vi "Example Read File.vi"() -> ()   [LabVIEW 2013]
uses:
  C:/tf/play/labview/Tinkerforge.dll
  Tinkerforge.dll
panel:
  out "transferred (byte)":i32
  in  "local path":path=path "C:/foobar.txt"
  in  "remote path":string="/home/tf/foobar.txt"
  in  "uid":string="XXYYZZ"
  in  "port":i32=4223
  in  "host":string="localhost"
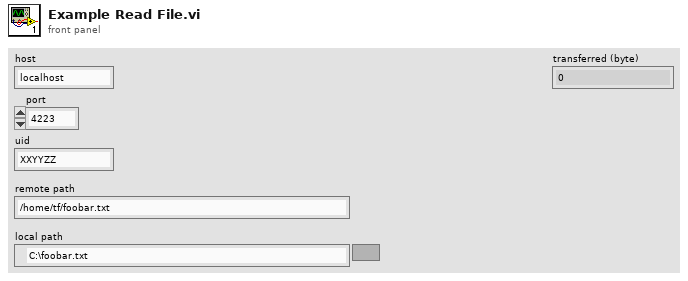
[diagram p1: front panel]
types:
  T1 = enum16{"open", "replace", "create", "open or create", "replace or create", "replace or create with confirmation"}
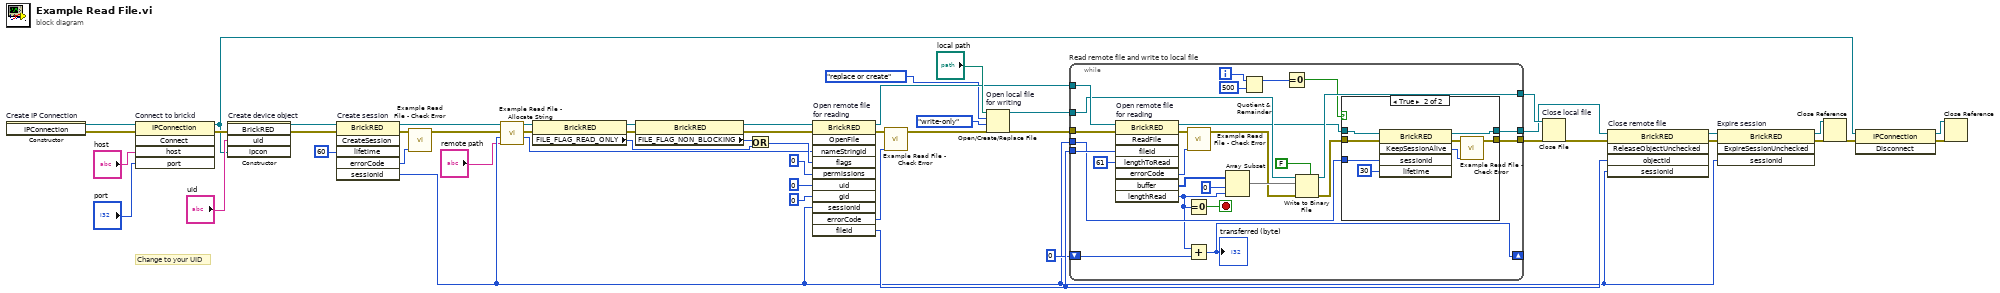
[diagram p0: block diagram]
diagram:
  # "Change to your UID"
  n1 = constructor on="Create IP Connection" class="IPConnection"() -> (reference out=w51:refnum<k24>, error out=w40:errorcluster)  [unwired: 3 in, 1 out]
  n2 = invoke on="Connect to brickd" class="IPConnection" method="Connect"(reference=w51, error in=w40, "host"="host", "port"="port") -> (reference out=w42:refnum<k24>, error out=w47:errorcluster)  [unwired: 1 in, 3 out]
  n3 = constructor on="Create device object" class="BrickRED"(error in=w47, "uid"="uid", "ipcon"=w42) -> (reference out=w45:refnum<k24>, error out=w46:errorcluster)  [unwired: 2 in, 3 out]
  n4 = invoke on="Create session" class="BrickRED" method="CreateSession"(reference=w45, error in=w46, "lifetime"=i64 60) -> (reference out=w6:refnum<k24>, error out=w38:errorcluster, "errorCode"=w37:u8, "sessionId"=w5:i32)  [unwired: 3 in, 2 out]
  n5 = call "Example Read File - Check Error.vi"("error code"=w37, "error in"=w38) -> ("error out"=w4:errorcluster)  [unwired: 9 in]
  n6 = call "Example Read File - Allocate String.vi"("buffer"="remote path", "session id"=w5, "error in"=w4, "reference in"=w6) -> ("string id"=w2:i32, "error out"=w3:errorcluster, "reference out"=w7:refnum<k24>)  [unwired: 5 in]
  n7 = property class="BrickRED"(reference=w7, error in=w3) -> (reference out=w28:refnum<k24>, error out=w31:errorcluster, "FILE_FLAG_READ_ONLY"=w26:i64)
  n8 = property class="BrickRED"(reference=w28, error in=w31) -> (reference out=w29:refnum<k24>, error out=w30:errorcluster, "FILE_FLAG_NON_BLOCKING"=w27:i64)
  n9 = Or(x=w27, y=w26) -> (x .or. y?=w25:i64)
  n10 = invoke on="Open remote file\nfor reading" class="BrickRED" method="OpenFile"(reference=w29, error in=w30, "nameStringId"=w2, "flags"=w25, "permissions"=0, "uid"=i64 0, "gid"=i64 0, "sessionId"=w5) -> (reference out=w20:refnum<k24>, error out=w35:errorcluster, "errorCode"=w36:u8, "fileId"=w16:i32)  [unwired: 3 in, 7 out]
  n11 = call "Example Read File - Check Error.vi"("error code"=w36, "error in"=w35) -> ("error out"=w23:errorcluster)  [unwired: 9 in]
  n12 = Open/Create/Replace File "Open local file\nfor writing"(file path (use dialog)="local path", error in=w23, operation (0:open)=T1."replace or create", access (0:read/write)=enum16{"read/write", "read-only", "write-only"}."write-only") -> (refnum out=w19:refnum<file>, error out=w21:errorcluster)  [unwired: 2 in, 1 out]
  n13 = while "Read remote file and write to local file" {
    tunnel: w21 -> [w77]
    tunnel: [w57] -> w18
    tunnel: w20 -> [w76]
    tunnel: [w59] -> w15
    tunnel: w16 -> [w75]
    tunnel: w19 -> [w71]
    tunnel: [w66] -> w17
    tunnel: w5 -> [w56]
    shift-right: [w53] -> _
    shift-left: 0 -> [w52]
    i -> [w64]
    stop <- w55 stop-if-true
    n14 = invoke on="Open remote file\nfor reading" class="BrickRED" method="ReadFile"(reference=w76, error in=w77, "fileId"=w75, "lengthToRead"=u8 61) -> (reference out=w60:refnum<k24>, error out=w72:errorcluster, "errorCode"=w73:u8, "buffer"=w70:u8[], "lengthRead"=w54:u8)  [unwired: 4 in, 3 out]
    n15 = Equal To 0?(x=w54) -> (x = 0?=w55:bool)
    n16 = Add(x=w54, y=w52) -> (x+y=w53:i32)
    "transferred (byte)" <- w53
    n17 = call "Example Read File - Check Error.vi"("error code"=w73, "error in"=w72) -> ("error out"=w67:errorcluster)  [unwired: 9 in]
    n18 = Array Subset(array=w70, index=0, length=w54) -> (w68:u8[])
    n19 = Quotient & Remainder(x=w64, y=500) -> (x-y*floor(x/y)=w62:i32)  [unwired: 1 out]
    n20 = Equal To 0?(x=w62) -> (x = 0?=w61:bool)
    n21 = Write to Binary File(file (use dialog)=w71, data=w68, error in=w67, 5:FALSE ("prepend array or string size? (T)")) -> (refnum out=w66:refnum<file>, error out=w58:errorcluster)  [unwired: 2 in, 1 out]
    n22 = case shown="True" w61 {
      tunnel: w60 -> [w79 w87]
      tunnel: [w79 w86] -> w59
      tunnel: w58 -> [w78 w85]
      tunnel: [w78 w80] -> w57
      tunnel: w56 -> [_ w84]
      frame False {
      }
      frame True {
        n23 = invoke class="BrickRED" method="KeepSessionAlive"(reference=w87, error in=w85, "sessionId"=w84, "lifetime"=i64 30) -> (reference out=w86:refnum<k24>, error out=w81:errorcluster, "KeepSessionAlive"=w82:u8)  [unwired: 1 in, 2 out]
        n24 = call "Example Read File - Check Error.vi"("error code"=w82, "error in"=w81) -> ("error out"=w80:errorcluster)  [unwired: 9 in]
      }
    }
  }
  n25 = Close File "Close local file"(refnum=w17, error in=w18) -> (error out=w14:errorcluster)  [unwired: 1 out]
  n26 = invoke on="Close remote file" class="BrickRED" method="ReleaseObjectUnchecked"(reference=w15, error in=w14, "objectId"=w16, "sessionId"=w5) -> (reference out=w12:refnum<k24>, error out=w13:errorcluster)  [unwired: 1 in, 3 out]
  n27 = invoke on="Expire session" class="BrickRED" method="ExpireSessionUnchecked"(reference=w12, error in=w13, "sessionId"=w5) -> (reference out=w11:refnum<k24>, error out=w10:errorcluster)  [unwired: 1 in, 2 out]
  n28 = Close Reference(reference=w11, error in (no error)=w10) -> (error out=w44:errorcluster)
  n29 = invoke class="IPConnection" method="Disconnect"(reference=w42, error in=w44) -> (reference out=w41:refnum<k24>, error out=w43:errorcluster)  [unwired: 1 in, 1 out]
  n30 = Close Reference(reference=w41, error in (no error)=w43) -> ()  [unwired: 1 out]
